vi "Get factory trim-9250.vi"(8 "error in (no error)":errorcluster, 11 "Accelerometer":T1) -> (0 "error out":errorcluster, 1 "Accel trim":dbl[](array[numeric]), 2 "Gyro trim":dbl[](array[numeric]), 3 "Accelerometer out":T1)   [LabVIEW 2013]
doc: "Use this template to build a VI to use as a subVI."
uses:
  AccelerometerSPI.ctl
  <vilib>/ni845x/ni845x.llb/ni845xControl.ctl
  <vilib>/ni845x/ni845x.llb/ni845xSpiConfiguration.ctl
  9250registers.ctl
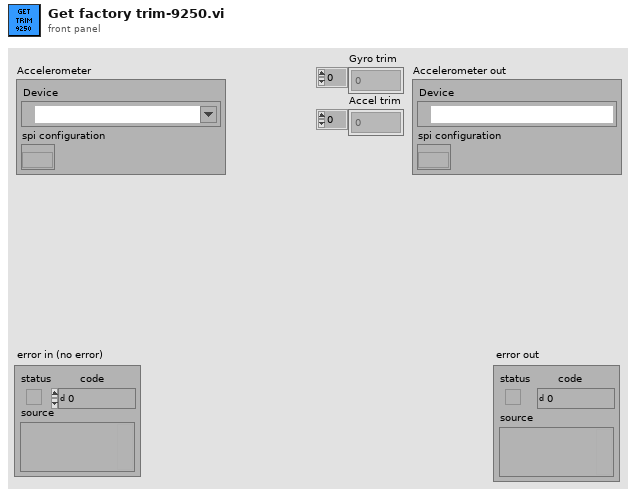
[diagram p1: front panel]
types:
  T1 = typedef "AccelerometerSPI.ctl" = cluster{"Device":T2, "spi configuration":T3}
  T2 = typedef "ni845xControl.ctl" = refnum<k21>
  T3 = typedef "ni845xSpiConfiguration.ctl" = refnum<k20>
  T4 = typedef "9250registers.ctl" = u8
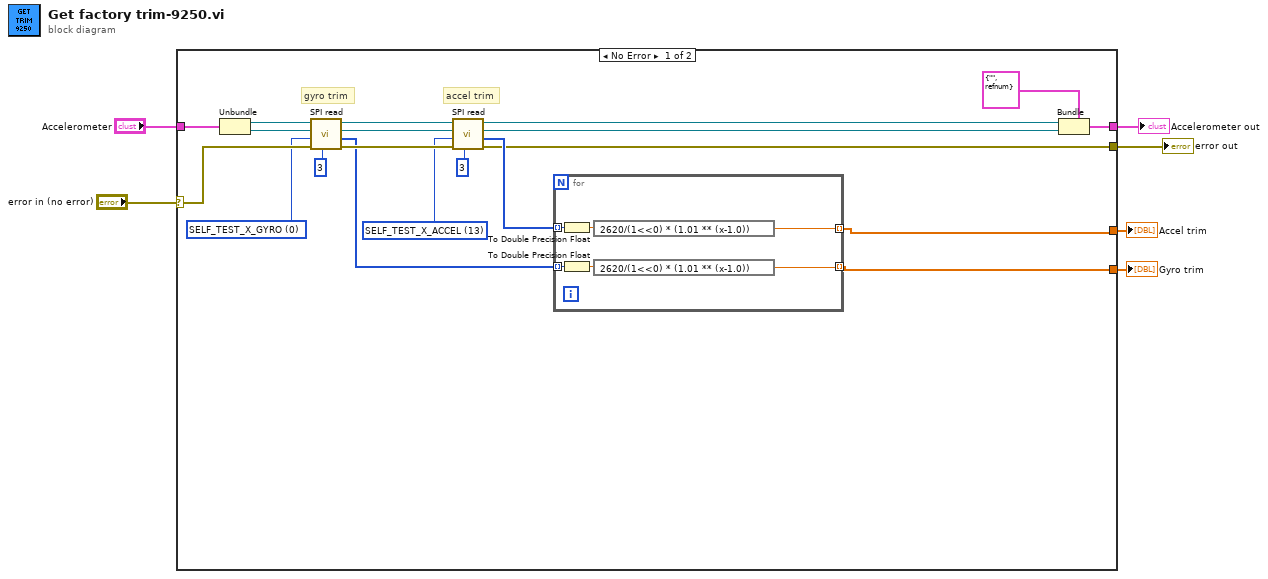
[diagram p0: block diagram]
diagram:
  n1 = case shown="No Error" "error in (no error)" {
    selector: "error in (no error)" -> [w23 w34]
    tunnel: [w9 w34] -> w5
    tunnel: "Accelerometer" -> [w26 w33]
    tunnel: [w20 w33] -> w3
    tunnel: [w12 _] -> w2
    tunnel: [w13 _] -> w1
    frame No Error {
      w7 = T4 13 items=["SELF_TEST_X_GYRO"=0, "SELF_TEST_Y_GYRO"=1, "SELF_TEST_Z_GYRO"=2, "SELF_TEST_X_ACCEL"=13, "SELF_TEST_Y_ACCEL"=14, "SELF_TEST_Z_ACCEL"=15, "XG_OFFSET"=19, "YG_OFFSET"=21, "ZG_OFFSET"=23, "SMPLRT_DIV"=25, "CONFIG"=26, "GYRO_CONFIG"=27, "ACCEL_CONFIG"=28, "ACCEL_CONFIG2"=29, "FIFO_EN"=35, "I2C_MST_CTRL"=36, "I2C_SLV0_ADDR"=37, "I2C_SLV0_REG"=38, "I2C_SLV0_CTRL"=39, "I2C_MST_STATUS"=54, "INT_ENABLE"=56, "INT_STATUS"=58, "ACCEL_XOUT"=59, "ACCEL_YOUT"=61, "ACCEL_ZOUT"=63, "TEMP_OUT"=65, "GYRO_XOUT"=67, "GYRO_YOUT"=69, "GYRO_ZOUT"=71, "EXT_SENS_DATA_00"=73, "I2C_SLV0_D0"=99, "USER_CTRL"=106, "PWR_MGMT_1"=107, "PWR_MGMT_2"=108, "WHO_AM_I"=117, "XA_OFFSET"=119, "YA_OFFSET"=122, "ZA_OFFSET"=125] ("9250 Registers")
      w8 = T4 0 items=["SELF_TEST_X_GYRO"=0, "SELF_TEST_Y_GYRO"=1, "SELF_TEST_Z_GYRO"=2, "SELF_TEST_X_ACCEL"=13, "SELF_TEST_Y_ACCEL"=14, "SELF_TEST_Z_ACCEL"=15, "XG_OFFSET"=19, "YG_OFFSET"=21, "ZG_OFFSET"=23, "SMPLRT_DIV"=25, "CONFIG"=26, "GYRO_CONFIG"=27, "ACCEL_CONFIG"=28, "ACCEL_CONFIG2"=29, "FIFO_EN"=35, "I2C_MST_CTRL"=36, "I2C_SLV0_ADDR"=37, "I2C_SLV0_REG"=38, "I2C_SLV0_CTRL"=39, "I2C_MST_STATUS"=54, "INT_ENABLE"=56, "INT_STATUS"=58, "ACCEL_XOUT"=59, "ACCEL_YOUT"=61, "ACCEL_ZOUT"=63, "TEMP_OUT"=65, "GYRO_XOUT"=67, "GYRO_YOUT"=69, "GYRO_ZOUT"=71, "EXT_SENS_DATA_00"=73, "I2C_SLV0_D0"=99, "USER_CTRL"=106, "PWR_MGMT_1"=107, "PWR_MGMT_2"=108, "WHO_AM_I"=117, "XA_OFFSET"=119, "YA_OFFSET"=122, "ZA_OFFSET"=125] ("9250 Registers")
      # "accel trim"
      # "gyro trim"
      n2 = Unbundle(w26) -> ("Device"=w25:T2, "spi configuration"=w24:T3)
      n3 = call "SPI read.vi"("Number of bytes"=3, "error in (no error)"=w23, "Address"=w8, "spi configuration in"=w24, "Device ref in"=w25) -> ("error out"=w16:errorcluster, "read data"=w14:u8[], "spi configuration out"=w17:T3, "Device ref out"=w18:T2)  [unwired: 3 in]
      n4 = call "SPI read.vi"("Number of bytes"=3, "error in (no error)"=w16, "Address"=w7, "spi configuration in"=w17, "Device ref in"=w18) -> ("error out"=w9:errorcluster, "read data"=w15:u8[], "spi configuration out"=w10:T3, "Device ref out"=w11:T2)  [unwired: 3 in]
      n5 = for {
        tunnel: w15 -> [w32] mode=indexing
        tunnel: [w31] -> w13 mode=indexing
        tunnel: w14 -> [w28] mode=indexing
        tunnel: [w27] -> w12 mode=indexing
        n6 = To Double Precision Float(number=w32) -> (double precision float=w30:dbl)
        n7 = To Double Precision Float(number=w28) -> (double precision float=w29:dbl)
        n8 = expression code="2620/(1<<0) * (1.01 ** (x-1.0))"(w30) -> (w31:dbl)
        n9 = expression code="2620/(1<<0) * (1.01 ** (x-1.0))"(w29) -> (w27:dbl)
      }
      n10 = Bundle(cluster=T1 {"Device"="", "spi configuration"=refnum} ("Accelerometer"), "Device"=w11, "spi configuration"=w10) -> (w20:T1)
    }
    frame Error {
    }
  }
  "error out" <- w5
  "Accelerometer out" <- w3
  "Gyro trim" <- w2
  "Accel trim" <- w1
